vi "PAQmem_ReadSection.vi"(6 "TagsIndices":i32[](array[numeric]), 8 "error in (no error)":errorcluster, 9 "Length":i32, 10 "Start":i32, 11 "PAQ-memory in":refnum<class "PAQ-memory.lvclass">) -> (0 "error out":errorcluster, 2 "DataSection":T1(array[cluster]), 3 "PAQ-memory out":refnum<class "PAQ-memory.lvclass">)   [LabVIEW 2020, in "PAQ-memory.lvclass"]
doc: "Andre Koelewijn, 17 jan 2021\n\nRead a section of the PAQ memory"
uses:
  PAQ-memory.lvclass
  PAQ-memory.lvclass/PAQ-memory.ctl
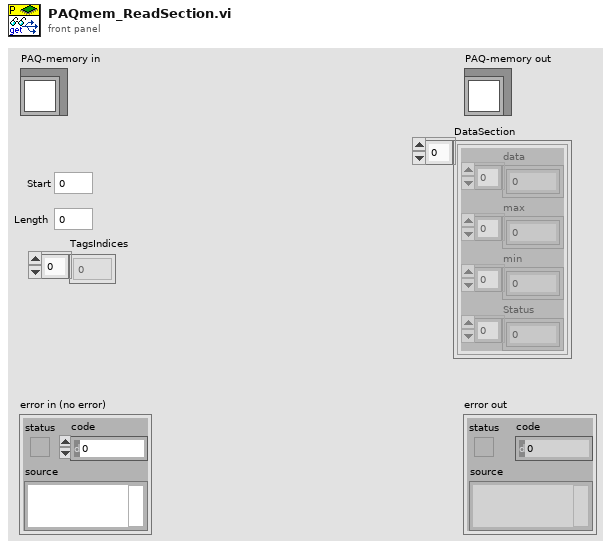
[diagram p1: front panel]
types:
  T1 = cluster{"data":dbl[], "max":dbl[], "min":dbl[], "Status":u32[]}[]
  T2 = cluster{"data":dbl[], "max":dbl[], "min":dbl[], "Status":u32[]}
  T3 = typedef "FAMM.lvclass/typedef_PAQdata.ctl" = cluster{"TAGs":string[], "Time":refnum<data-value>, "TAGdata":cluster{"source":refnum<data-value>, "status":refnum<data-value>, "data":refnum<data-value>, "max":refnum<data-value>, "min":refnum<data-value>}[]}
  T4 = cluster{"source":refnum<data-value>, "status":refnum<data-value>, "data":refnum<data-value>, "max":refnum<data-value>, "min":refnum<data-value>}[]
  T5 = cluster{"source":refnum<data-value>, "status":refnum<data-value>, "data":refnum<data-value>, "max":refnum<data-value>, "min":refnum<data-value>}
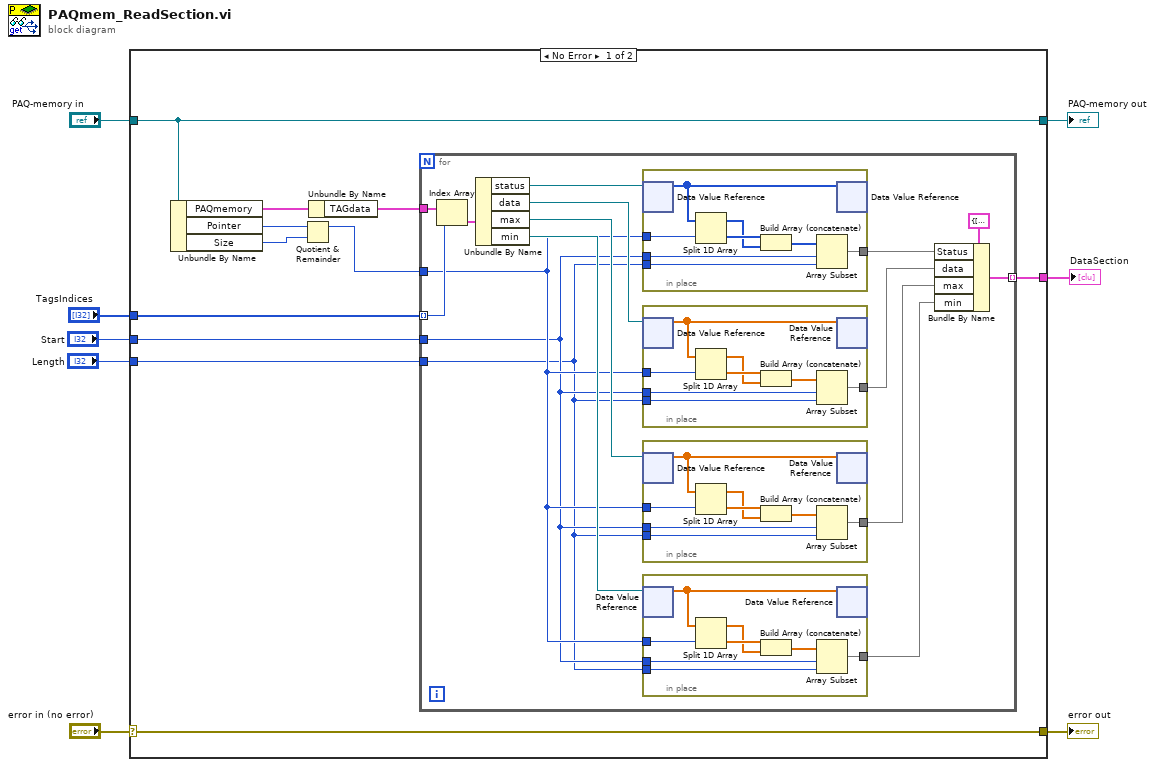
[diagram p0: block diagram]
diagram:
  n1 = case shown="No Error" "error in (no error)" {
    selector: "error in (no error)" -> [w10 w69]
    tunnel: [w10 w69] -> w7
    tunnel: [w11 w68] -> w5
    tunnel: "PAQ-memory in" -> [w11 w68]
    tunnel: "TagsIndices" -> [w15 _]
    tunnel: "Start" -> [w13 _]
    tunnel: "Length" -> [w12 _]
    tunnel: [w9 _] -> w1
    frame No Error {
      n2 = Unbundle By Name(w11) -> ("PAQmemory"=w19:T3, "Pointer"=w17:i32, "Size"=w16:i32)
      n3 = Quotient & Remainder(x=w17, y=w16) -> (x-y*floor(x/y)=w18:i32)  [unwired: 1 out]
      n4 = Unbundle By Name(w19) -> ("TAGdata"=w14:T4)
      n5 = for {
        tunnel: w18 -> [w28]
        tunnel: w15 -> [w34] mode=indexing
        tunnel: w14 -> [w35]
        tunnel: w13 -> [w27]
        tunnel: w12 -> [w26]
        tunnel: [w20] -> w9 mode=indexing
        n6 = Index Array(array=w35, index=w34) -> (element=w33:T5)
        n7 = Unbundle By Name(w33) -> ("status"=w32:refnum<data-value>, "data"=w31:refnum<data-value>, "max"=w30:refnum<data-value>, "min"=w29:refnum<data-value>)
        n8 = in-place {
          in-place-border: w28 -> [w66]
          in-place-border: w27 -> [w62]
          in-place-border: w26 -> [w61]
          in-place-border: [w60] -> w24
          n9 = in-place-dvr #1(w32) -> (w67:u32[])  [unwired: 1 out]
          n10 = Split 1D Array(array=w67, index=w66) -> (first subarray=w64:u32[], second subarray=w65:u32[])
          n11 = Build Array (concatenate)(w65, w64) -> (w63:u32[])
          n12 = Array Subset(array=w63, index=w62, length=w61) -> (w60:u32[])
          n13 = in-place-dvr #1(w67) -> ()  [unwired: 2 out]
        }
        n14 = in-place {
          in-place-border: w28 -> [w58]
          in-place-border: w27 -> [w54]
          in-place-border: w26 -> [w53]
          in-place-border: [w52] -> w23
          n15 = in-place-dvr #2(w31) -> (w59:dbl[])  [unwired: 1 out]
          n16 = Split 1D Array(array=w59, index=w58) -> (first subarray=w56:dbl[], second subarray=w57:dbl[])
          n17 = Build Array (concatenate)(w57, w56) -> (w55:dbl[])
          n18 = Array Subset(array=w55, index=w54, length=w53) -> (w52:dbl[])
          n19 = in-place-dvr #2(w59) -> ()  [unwired: 2 out]
        }
        n20 = in-place {
          in-place-border: w28 -> [w50]
          in-place-border: w27 -> [w46]
          in-place-border: w26 -> [w45]
          in-place-border: [w44] -> w22
          n21 = in-place-dvr #3(w30) -> (w51:dbl[])  [unwired: 1 out]
          n22 = Split 1D Array(array=w51, index=w50) -> (first subarray=w48:dbl[], second subarray=w49:dbl[])
          n23 = Build Array (concatenate)(w49, w48) -> (w47:dbl[])
          n24 = Array Subset(array=w47, index=w46, length=w45) -> (w44:dbl[])
          n25 = in-place-dvr #3(w51) -> ()  [unwired: 2 out]
        }
        n26 = in-place {
          in-place-border: w28 -> [w42]
          in-place-border: w27 -> [w38]
          in-place-border: w26 -> [w37]
          in-place-border: [w36] -> w21
          n27 = in-place-dvr #4(w29) -> (w43:dbl[])  [unwired: 1 out]
          n28 = Split 1D Array(array=w43, index=w42) -> (first subarray=w40:dbl[], second subarray=w41:dbl[])
          n29 = Build Array (concatenate)(w41, w40) -> (w39:dbl[])
          n30 = Array Subset(array=w39, index=w38, length=w37) -> (w36:dbl[])
          n31 = in-place-dvr #4(w43) -> ()  [unwired: 2 out]
        }
        n32 = Bundle By Name(cluster=T2 {"data"=[], "max"=[], "min"=[], "Status"=[]} ("DataSection"), "Status"=w24, "data"=w23, "max"=w22, "min"=w21) -> (w20:T2)
      }
    }
    frame Error {
    }
  }
  "error out" <- w7
  "PAQ-memory out" <- w5
  "DataSection" <- w1
